vi "CAL-Save data.vi"(0 "Mag":dbl[](array[numeric]), 1 "backup":bool=TRUE, 5 "Phase":dbl[](array[numeric]), 7 "Frequency":dbl[](array[numeric]), 9 "path":path, 11 "error in (no error)":errorcluster, 12 "Cal Stimulus":T1={"Min Freq (Hz)"=50.0, "Max Freq (Hz)"=50000.0, "Freq Step (Hz)"=50.0, "Waveform"=enum."Chirp", "Attenuation (dB)"=20.0, "Sample Rate (Hz)"=100000.0}, 13 "Probe Tube File":path) -> (6 "new file path":path, 15 "error out":errorcluster)   [LabVIEW 2020]
uses:
  In-Ear Calibration VIs/LV Source/Type Defs/Cal Stimulus.ctl
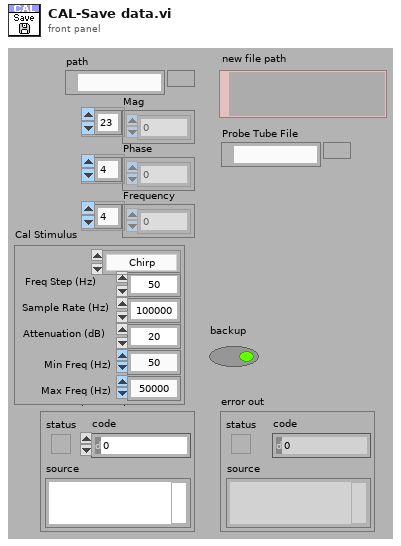
[diagram p1: front panel]
types:
  T1 = typedef "Cal Stimulus.ctl" = cluster{"Min Freq (Hz)":dbl, "Max Freq (Hz)":dbl, "Freq Step (Hz)":dbl, "Waveform":enum16{"Chirp", "Weighted"}, "Attenuation (dB)":dbl, "Sample Rate (Hz)":dbl}
  T2 = enum16{"open", "replace", "create", "open or create", "replace or create", "replace or create with confirmation"}
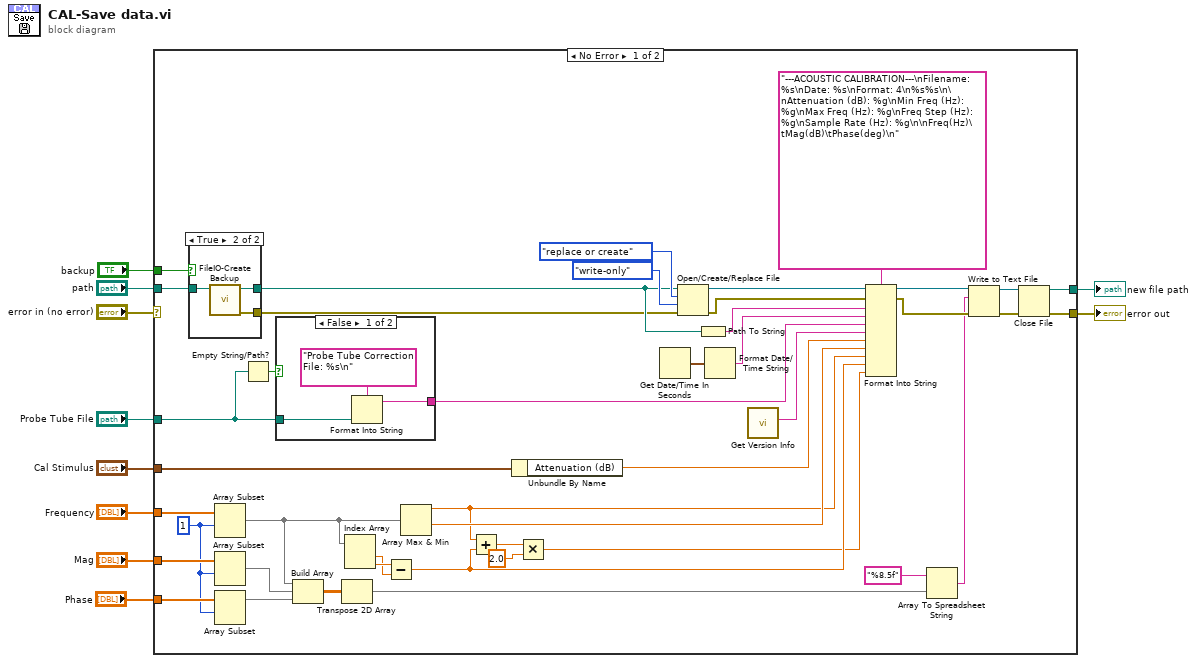
[diagram p0: block diagram]
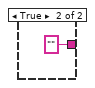
[diagram p3: hidden frame]
diagram:
  n1 = case shown="No Error" "error in (no error)" {
    selector: "error in (no error)" -> [_ w62]
    tunnel: "Phase" -> [w53 _]
    tunnel: "Mag" -> [w52 _]
    tunnel: "Frequency" -> [w32 _]
    tunnel: [w38 w62] -> w7
    tunnel: "Cal Stimulus" -> [w50 _]
    tunnel: [w37 _] -> w4
    tunnel: "path" -> [w14 _]
    tunnel: "Probe Tube File" -> [w30 _]
    tunnel: "backup" -> [w11 _]
    frame No Error {
      w27 = 1 ("index")
      n2 = case shown="True" w11 {
        tunnel: w14 -> [w54 w57]
        tunnel: [w54 w56] -> w13
        tunnel: [_ w55] -> w12
        frame False {
        }
        frame True {
          n3 = call "FileIO-Create Backup.vi"("Path"=w57) -> ("error out"=w55:errorcluster, "Path (thru)"=w56:path)  [unwired: 7 in, 2 out]
        }
      }
      n4 = Array Subset(array=w32, index=w27) -> (w25:dbl[])  [unwired: 1 in]
      n5 = Array Subset(array=w52, index=w27) -> (w29:dbl[])  [unwired: 1 in]
      n6 = Array Subset(array=w53, index=w27) -> (w28:dbl[])  [unwired: 1 in]
      n7 = Empty String/Path?(string/path=w30) -> (empty?=w31:bool)
      n8 = case shown="False" w31 {
        tunnel: w30 -> [w59 _]
        tunnel: [w58 ""] -> w17
        frame False {
          n9 = Format Into String(format string="Probe Tube Correction File: %s\n", w59) -> (resulting string=w58:string)  [unwired: 2 in, 1 out]
        }
        frame True {
        }
      }
      n10 = Build Array(w25, w29, w28) -> (w45:dbl[][])
      n11 = Transpose 2D Array(2D array=w45) -> (transposed array=w44:dbl[][])
      n12 = Index Array(array=w25) -> (element #1=w23:dbl, element #2=w24:dbl)  [unwired: 2 in]
      n13 = Subtract(x=w24, y=w23) -> (x-y=w21:dbl)
      n14 = Array Max & Min(array=w25) -> (max value=w22:dbl, min value=w26:dbl)  [unwired: 2 out]
      n15 = Add(x=w22, y=w21) -> (x+y=w20:dbl)
      n16 = Unbundle By Name(w50) -> ("Attenuation (dB)"=w15:dbl)
      n17 = Multiply(x=w20, y=2.0) -> (x*y=w18:dbl)
      n18 = Get Date/Time In Seconds() -> (seconds since 1Jan1904=w48:timestamp)
      n19 = Open/Create/Replace File(file path (use dialog)=w13, error in=w12, operation (0:open)=T2."replace or create", access (0:read/write)=enum16{"read/write", "read-only", "write-only"}."write-only") -> (refnum out=w36:refnum<file>, error out=w33:errorcluster)  [unwired: 2 in, 1 out]
      n20 = Path To String(path=w13) -> (string=w49:string)
      n21 = Format Date/Time String(seconds (now)=w48) -> (date/time string=w47:string)  [unwired: 2 in]
      n22 = call "Get Version Info.vi"() -> ("Version Info"=w16:string)  [unwired: 11 in]
      n23 = Format Into String(format string="---ACOUSTIC CALIBRATION---\nFilename: %s\nDate: %s\nFormat: 4\n%s%s\n\nAttenuation (dB): %g\nMin Freq (Hz): %g\nMax Freq (Hz): %g\nFreq Step (Hz): %g\nSample Rate (Hz): %g\n\nFreq(Hz)\tMag(dB)\tPhase(deg)\n", initial string=w36, error in=w33, w49, w47, w17, w16, w15, w26, w22, w21, w18) -> (resulting string=w43:refnum<file>, error out=w42:errorcluster)
      n24 = Array To Spreadsheet String(array=w44, 3:"%8.5f" ("format (%.3f)")) -> (spreadsheet string=w41:string)  [unwired: 1 in]
      n25 = Write to Text File(file (use dialog)=w43, text=w41, error in=w42) -> (refnum out=w39:refnum<file>, error out=w40:errorcluster)  [unwired: 1 in, 1 out]
      n26 = Close File(refnum=w39, error in=w40) -> (path=w37:path, error out=w38:errorcluster)
    }
    frame Error {
    }
  }
  "error out" <- w7
  "new file path" <- w4
